vi "PostResults.vi"(0 "reference in":refnum<class "MES_Local.lvclass">, 11 "error in (no error)":errorcluster) -> (4 "reference in":refnum<class "MES_Local.lvclass">, 6 "Status":T1, 15 "error out":errorcluster)   [LabVIEW 2022 SP3, in "MES_Local.lvlib" / "MES_Local.lvclass"]
uses:
  MES_Local.lvclass
  Components/MES_Base.lvlibp/Controls/Status.ctl
  Components/MES_Base.lvlibp/MES_Base.lvclass
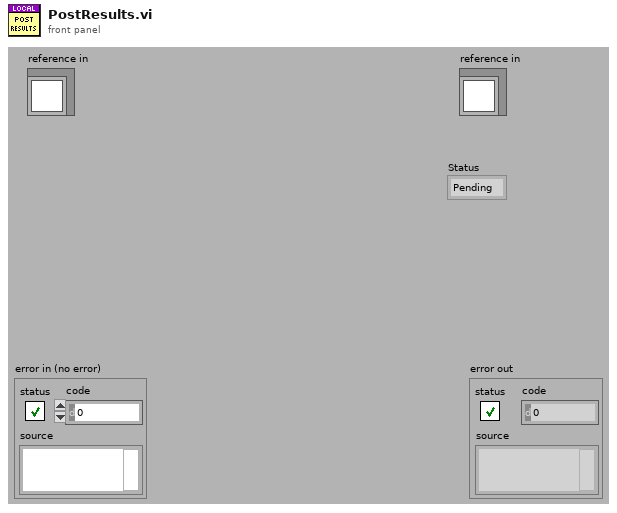
[diagram p1: front panel]
types:
  T1 = typedef "MES_Base.lvlibp/MES_Base.lvclass/Status.ctl" = enum16{"Pending", "Pass", "Fail"}
  T2 = typedef "MES_Local.lvlib/MES_Local.lvclass/ObjectAttributes.ctl" = cluster{"Config":T3, "Logged_In?":bool, "AttributeNames":string[], "AttributeWritten":bool[], "ComponentNames":string[], "TestIndex":i32, "TestTag":string[], "Time Stamp":timestamp, "Employee":string, "Resource_Key":string, "Local Spec":path, "Login":refnum<class "Login_Base.lvclass">, "ReportPath":path, "Spec":T4, "StartTime":timestamp, "Role":string}
  T3 = typedef "MES_Local.lvlib/MES_Local.lvclass/Config.ctl" = cluster{"Results_Path":path}
  T4 = typedef "MES_Base.lvlibp/MES_Base.lvclass/Spec.ctl" = cluster{"Header":cluster{"Doctype":string, "Checksum":string, "DriverKey":string, "SpecId":string, "TransactionId":string, "AccountId":string, "SpecName":string, "WorkflowStep":string, "SerialNumber":string, "BatchNumber":string, "Status":enum16{"Pending", "Pass", "Fail"}, "Comment":string, "FirstFail":string, "Employee":string, "LocalMachine":string, "ResourceKey":string, "Date":string, "Time":string, "Duration":string, "DUT Position":i32}, "Components":cluster{"SerialNumber":string, "PartNumber":string, "Revision":string, "BatchNumber":string, "Name":string, "Description":string, "Attached":bool}[], "Attributes":cluster{"Name":string, "Description":string, "DataType":enum16{"NA", "String", "Boolean", "Int", "Dbl"}, "Value":variant, "DisplayFormat":string, "ReadOnly":bool, "Required":bool}[], "Tests":cluster{"Code":string, "Name":string, "Description":string, "Group":string, "IsGroup":bool, "Tag":string, "Method":string, "Parrameter":string, "DataType":enum16{"NA", "String", "Boolean", "Int", "Dbl"}, "Value":variant, "Status":enum16{"Pending", "Pass", "Fail"}, "LimitLo":variant, "LimitHi":variant, "StringMatch":string, "BooleanMatch":bool, "DisplayFormat":string, "Units":string, "TestTime":dbl}[]}
  T5 = cluster{"Code":string, "Name":string, "Description":string, "Group":string, "IsGroup":bool, "Tag":string, "Method":string, "Parrameter":string, "DataType":enum16{"NA", "String", "Boolean", "Int", "Dbl"}, "Value":variant, "Status":enum16{"Pending", "Pass", "Fail"}, "LimitLo":variant, "LimitHi":variant, "StringMatch":string, "BooleanMatch":bool, "DisplayFormat":string, "Units":string, "TestTime":dbl}[]
  T6 = cluster{"SerialNumber":string, "PartNumber":string, "Revision":string, "BatchNumber":string, "Name":string, "Description":string, "Attached":bool}[]
  T7 = cluster{"Name":string, "Description":string, "DataType":enum16{"NA", "String", "Boolean", "Int", "Dbl"}, "Value":variant, "DisplayFormat":string, "ReadOnly":bool, "Required":bool}[]
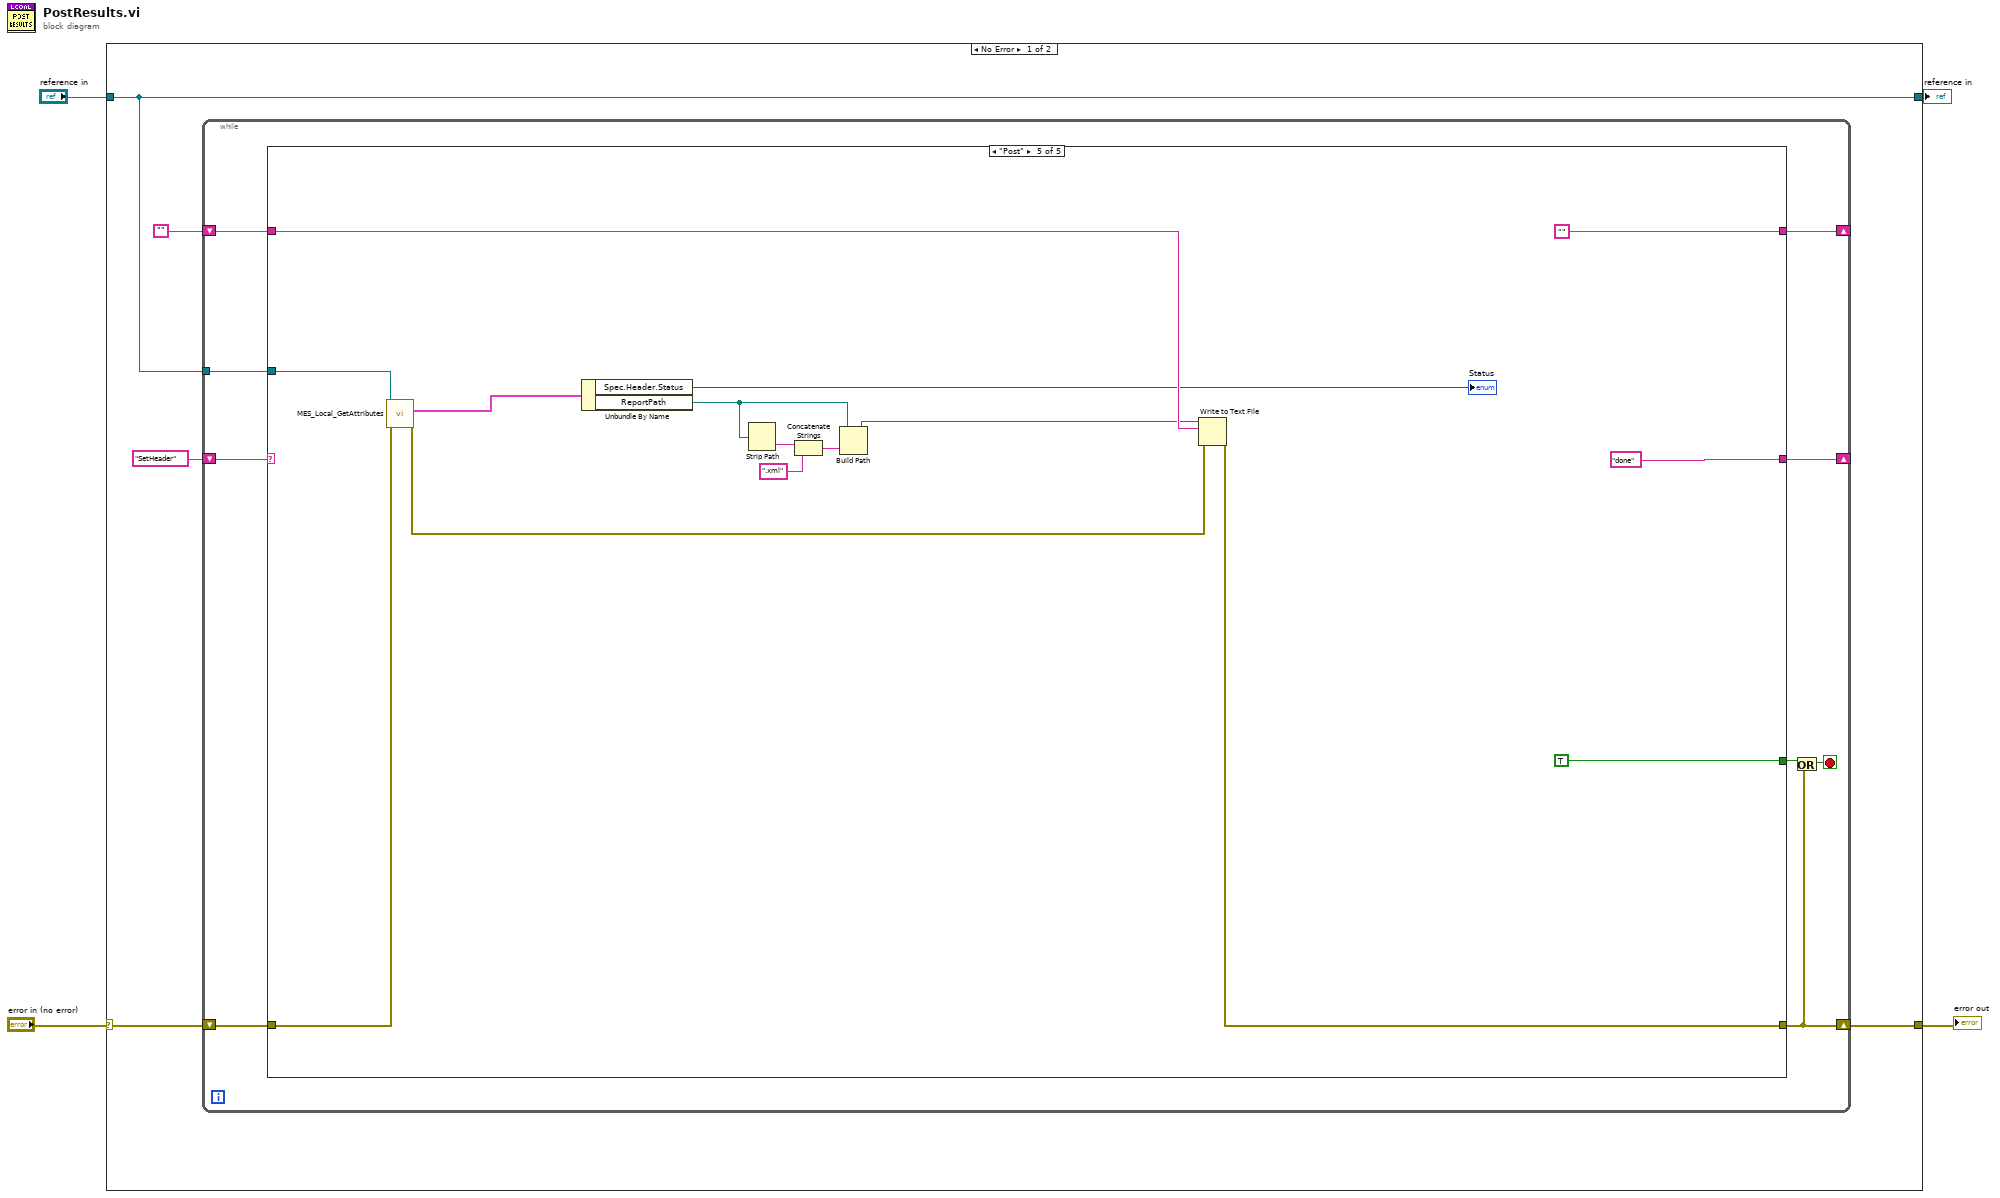
[diagram p0: block diagram]
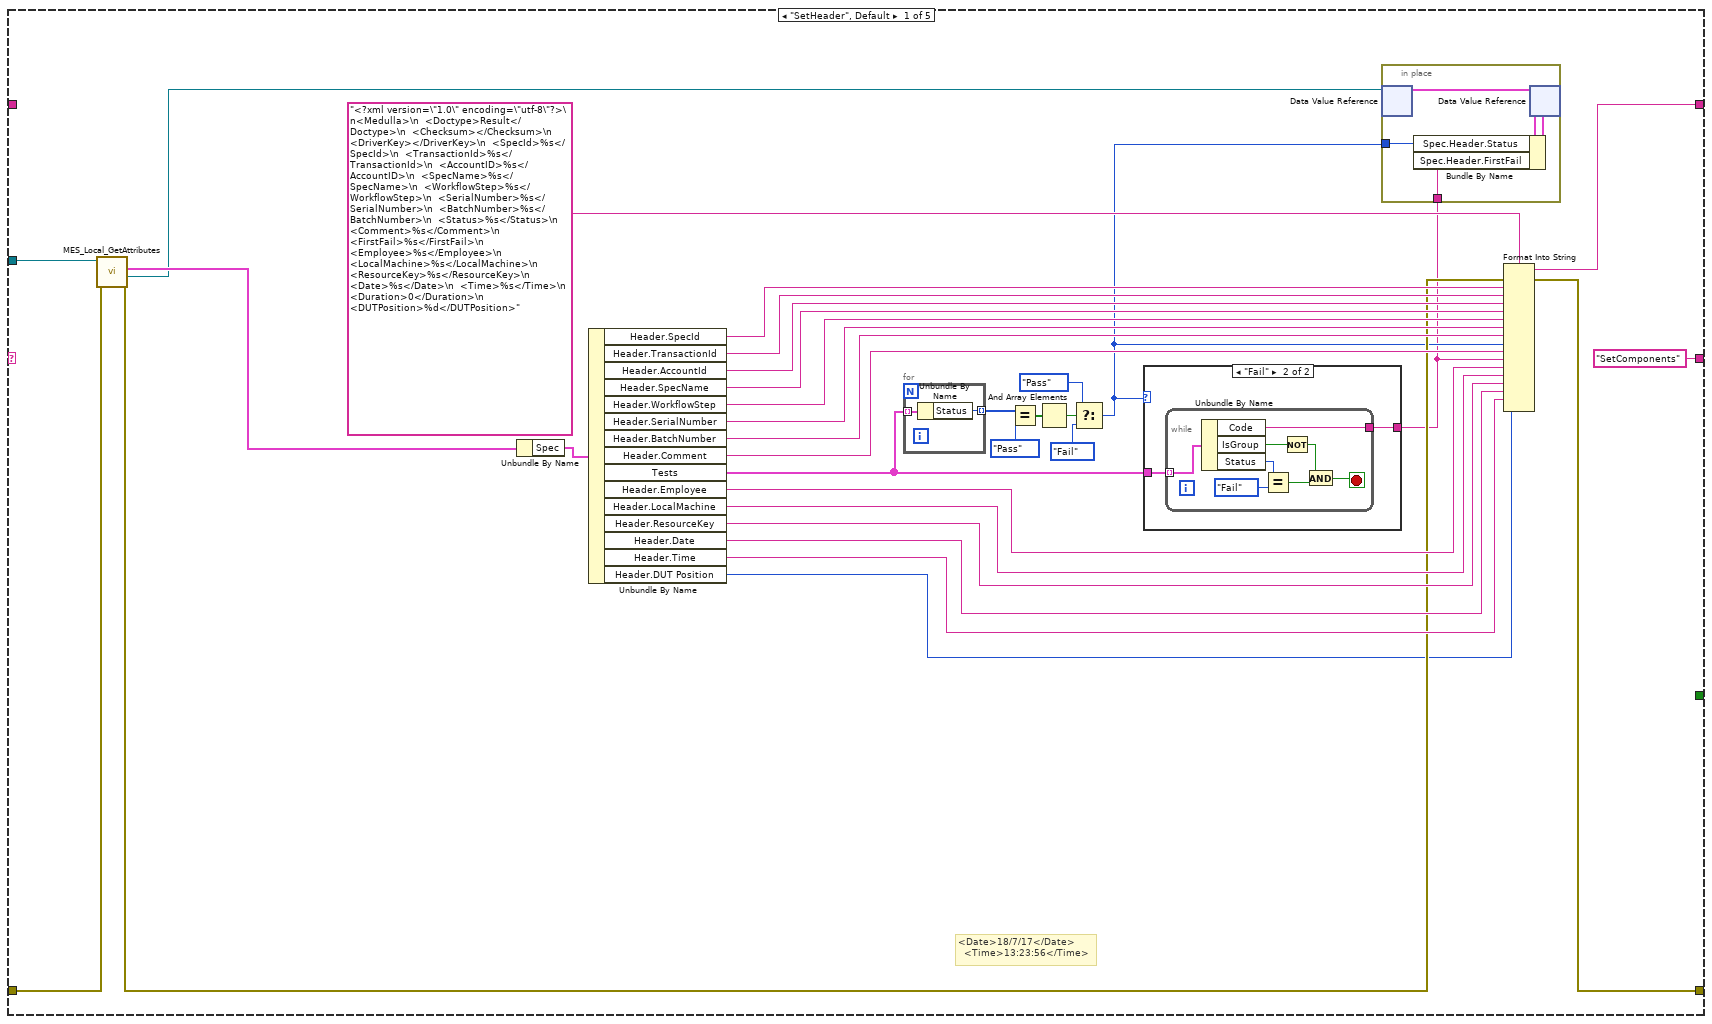
[diagram p2: hidden frame]
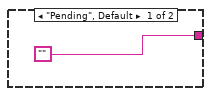
[diagram p3: hidden frame]
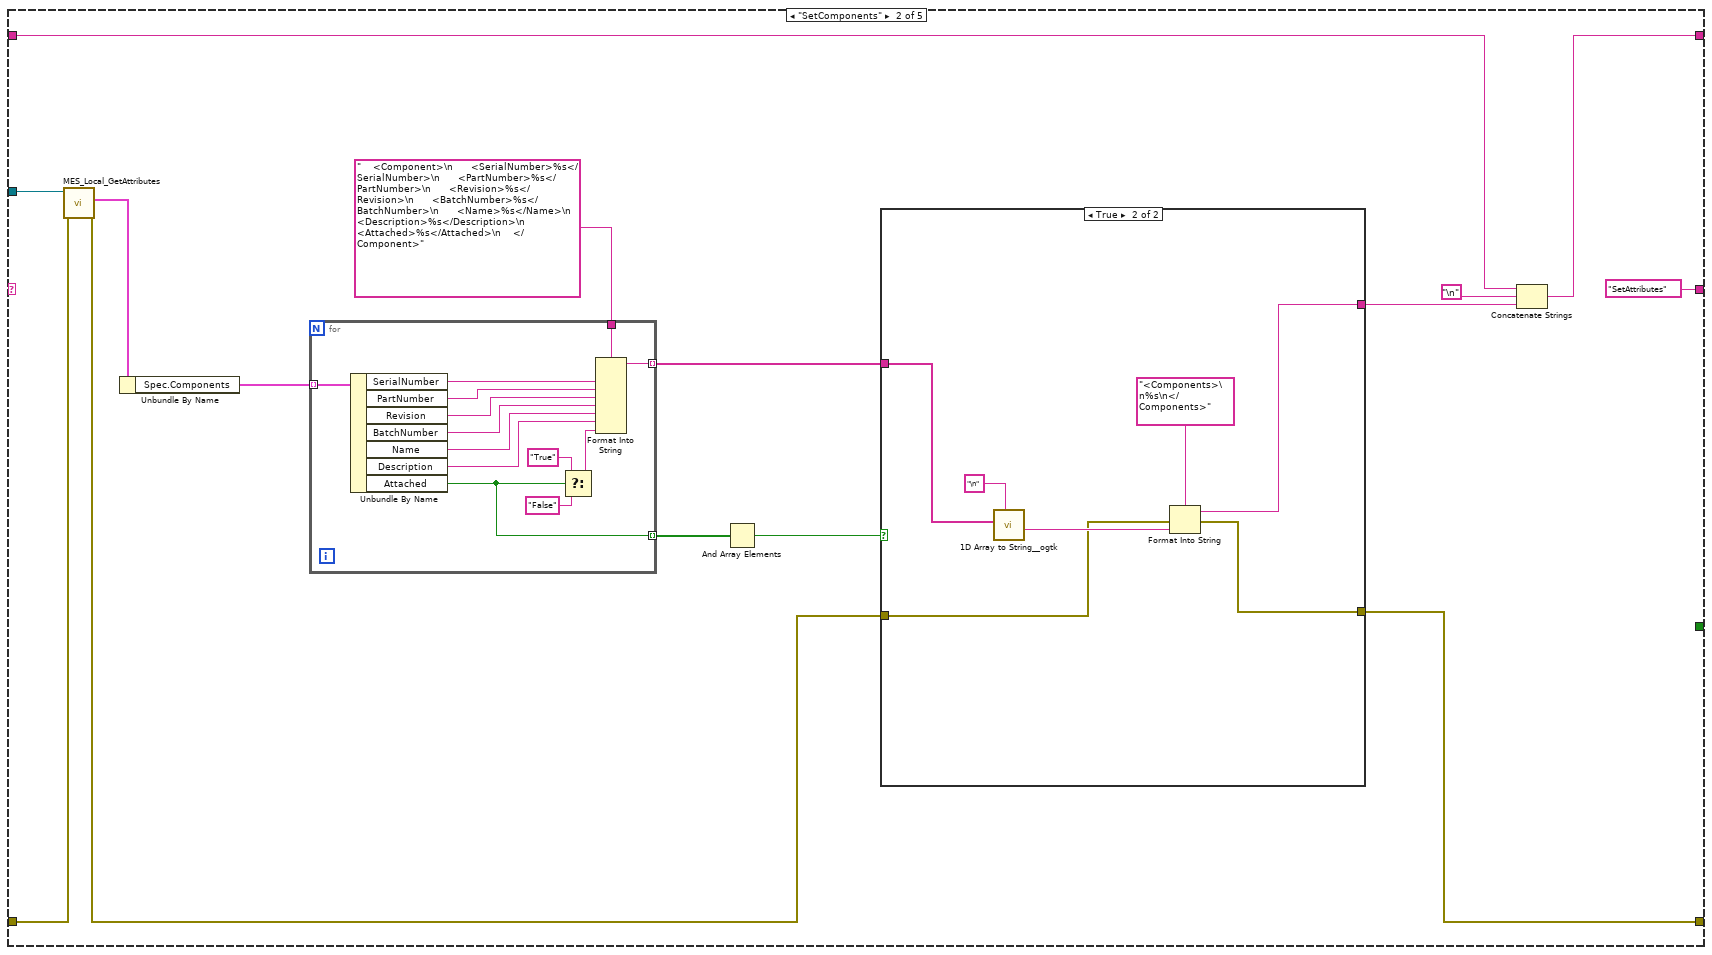
[diagram p4: hidden frame]
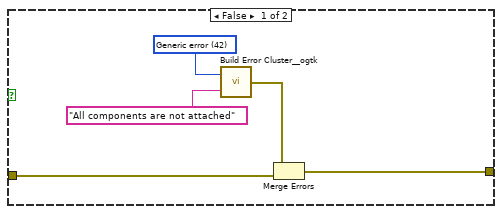
[diagram p5: hidden frame]
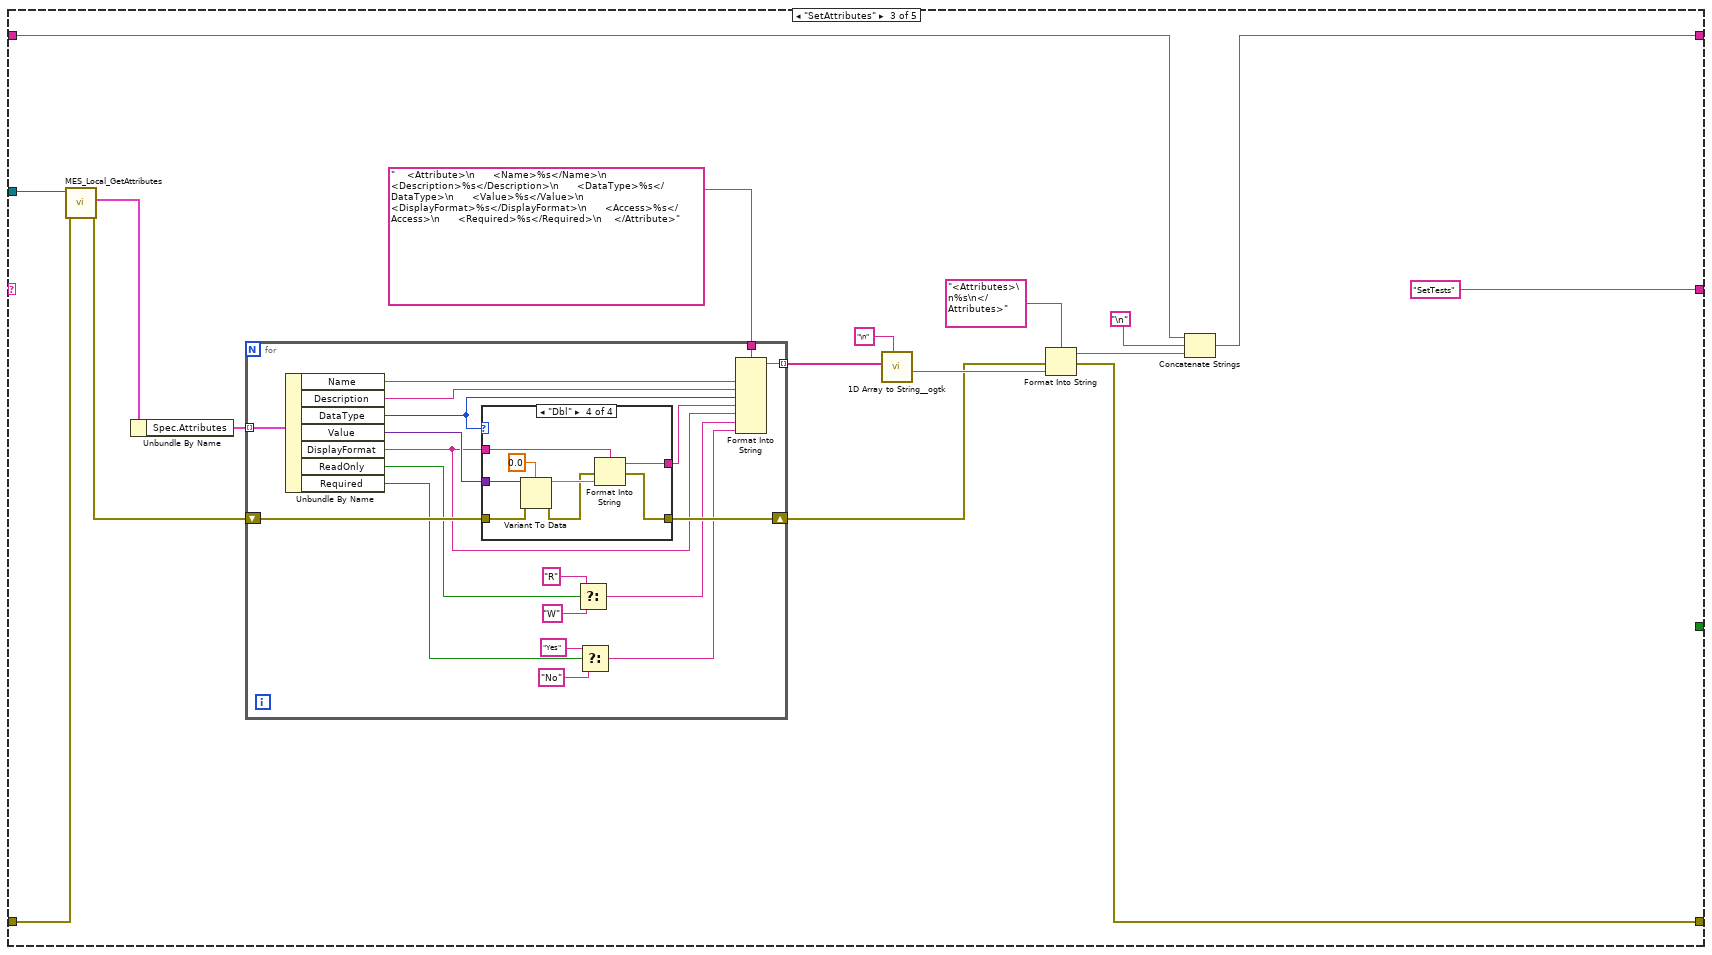
[diagram p6: hidden frame]
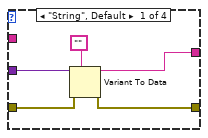
[diagram p7: hidden frame]
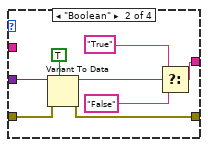
[diagram p8: hidden frame]
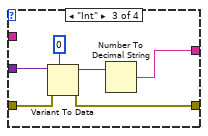
[diagram p9: hidden frame]
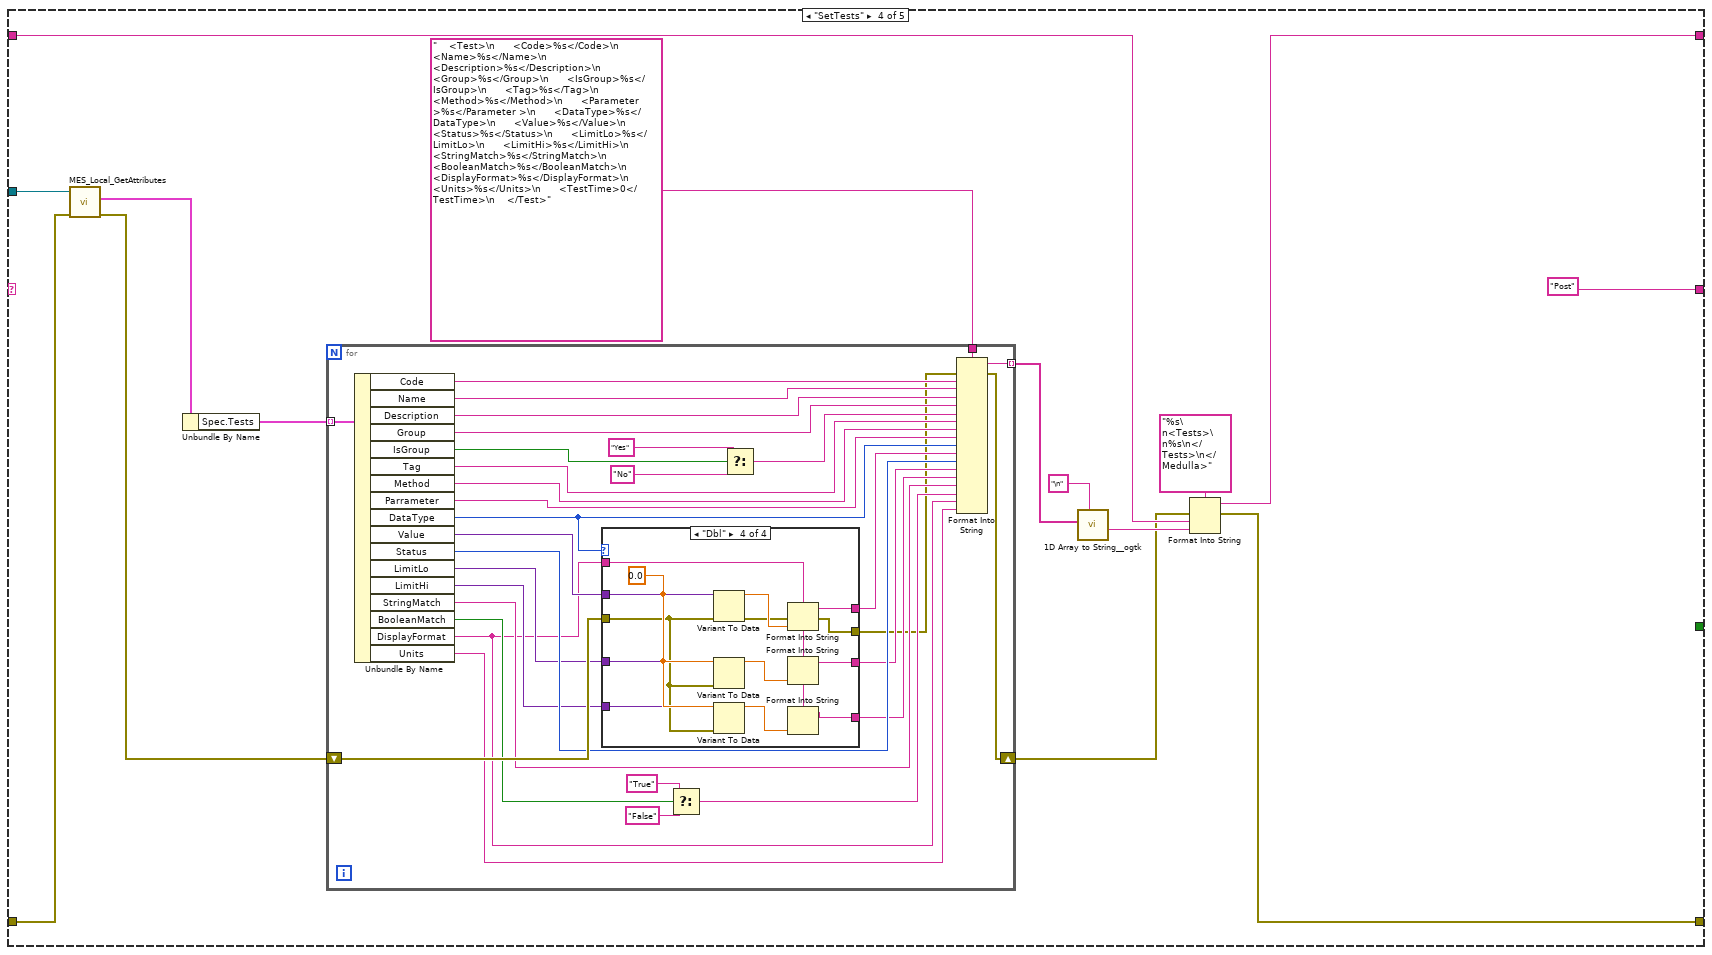
[diagram p10: hidden frame]
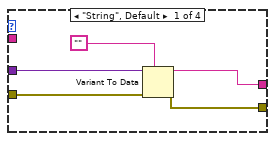
[diagram p11: hidden frame]
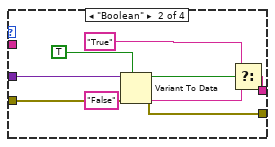
[diagram p12: hidden frame]
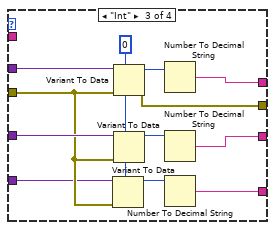
[diagram p13: hidden frame]
diagram:
  n1 = case shown="No Error" "error in (no error)" {
    selector: "error in (no error)" -> [w5 w274]
    tunnel: [w7 w274] -> w3
    tunnel: [w6 w273] -> w1
    tunnel: "reference in" -> [w6 w273]
    frame No Error {
      n2 = while {
        shift-right: [w12] -> _
        shift-left: "SetHeader" -> [w18]
        shift-right: [w16] -> w7
        shift-left: w5 -> [w17]
        shift-right: [w13] -> _
        shift-left: "" -> [w14]
        tunnel: w6 -> [w10]
        stop <- w15 stop-if-true
        n3 = case shown="\"Post\"" w18 {
          tunnel: w17 -> [w28 w71 w111 w173 w267]
          tunnel: [w51 w78 w122 w184 w269] -> w16
          tunnel: w14 -> [_ w76 w117 w183 w268]
          tunnel: [w47 w74 w115 w182 ""] -> w13
          tunnel: ["SetComponents" ("String to Prepend to source (\"\")") "SetAttributes" ("String to Prepend to source (\"\")") "SetTests" ("String to Prepend to source (\"\")") "Post" ("String to Prepend to source (\"\")") "done" ("String to Prepend to source (\"\")")] -> w12
          tunnel: [_ _ _ _ TRUE] -> w11
          tunnel: w10 -> [w29 w72 w112 w175 w266]
          frame "SetHeader", Default {
            # "<Date>18/7/17</Date>\n  <Time>13:23:56</Time>"
            n4 = call "MES_Local_GetAttributes.vi"("error in (no error)"=w28, "reference in"=w29) -> ("error out"=w27:errorcluster, "DataRef"=w25:refnum<data-value>, "Data"=w26:T2)  [unwired: 6 in, 1 out]
            n5 = Unbundle By Name(w26) -> ("Spec"=w48:T4)
            n6 = Unbundle By Name(w48) -> ("Header.SpecId"=w42:string, "Header.TransactionId"=w41:string, "Header.AccountId"=w40:string, "Header.SpecName"=w39:string, "Header.WorkflowStep"=w38:string, "Header.SerialNumber"=w37:string, "Header.BatchNumber"=w36:string, "Header.Comment"=w35:string, "Tests"=w49:T5, "Header.Employee"=w34:string, "Header.LocalMachine"=w33:string, "Header.ResourceKey"=w32:string, "Header.Date"=w31:string, "Header.Time"=w30:string, "Header.DUT Position"=w19:i32)
            n7 = for {
              tunnel: w49 -> [w68] mode=indexing
              tunnel: [w67] -> w50 mode=indexing
              n8 = Unbundle By Name(w68) -> ("Status"=w67:enum16{"Pending", "Pass", "Fail"})
            }
            n9 = Equal?(x=w50, y=Status."Pass" ("Status")) -> (x = y?=w44:bool[])
            n10 = And Array Elements(Boolean array=w44) -> (logical AND=w43:bool)
            n11 = Select(t=Status."Pass" ("Status"), s=w43, f=Status."Fail" ("Status")) -> (s? t:f=w24:T1)
            n12 = case shown="\"Fail\"" w24 {
              tunnel: ["" w57] -> w23
              tunnel: w49 -> [_ w58]
              frame "Pending", Default {
              }
              frame "Fail" {
                n13 = while {
                  tunnel: w58 -> [w66] mode=indexing
                  tunnel: [w60] -> w57
                  stop <- w61 stop-if-true
                  n14 = Unbundle By Name(w66) -> ("Code"=w60:string, "IsGroup"=w65:bool, "Status"=w64:enum16{"Pending", "Pass", "Fail"})
                  n15 = Equal?(x=w64, y=Status."Fail" ("Status")) -> (x = y?=w62:bool)
                  n16 = Not(x=w65) -> (.not. x?=w63:bool)
                  n17 = And(x=w63, y=w62) -> (x .and. y?=w61:bool)
                }
              }
            }
            n18 = in-place {
              in-place-border: w24 -> [w53]
              in-place-border: w23 -> [w52]
              n19 = in-place-dvr #1(w25) -> (w55:T2)  [unwired: 1 out]
              n20 = Bundle By Name(cluster=w55, "Spec.Header.Status"=w53, "Spec.Header.FirstFail"=w52) -> (w54:T2)
              n21 = in-place-dvr #1(w54) -> ()  [unwired: 2 out]
            }
            n22 = Format Into String(format string="<?xml version=\"1.0\" encoding=\"utf-8\"?>\n<Medulla>\n  <Doctype>Result</Doctype>\n  <Checksum></Checksum>\n  <DriverKey></DriverKey>\n  <SpecId>%s</SpecId>\n  <TransactionId>%s</TransactionId>\n  <AccountID>%s</AccountID>\n  <SpecName>%s</SpecName>\n  <WorkflowStep>%s</WorkflowStep>\n  <SerialNumber>%s</SerialNumber>\n  <BatchNumber>%s</BatchNumber>\n  <Status>%s</Status>\n  <Comment>%s</Comment>\n  <FirstFail>%s</FirstFail>\n  <Employee>%s</Employee>\n  <LocalMachine>%s</LocalMachine>\n  <ResourceKey>%s</ResourceKey>\n  <Date>%s</Date>\n  <Time>%s</Time>\n  <Duration>0</Duration>\n <DUTPosition>%d</DUTPosition>", error in=w27, w42, w41, w40, w39, w38, w37, w36, w24, w35, w23, w34, w33, w32, w31, w30, w19) -> (resulting string=w47:string, error out=w51:errorcluster)  [unwired: 1 in]
          }
          frame "SetComponents" {
            n23 = call "MES_Local_GetAttributes.vi"("error in (no error)"=w71, "reference in"=w72) -> ("error out"=w70:errorcluster, "Data"=w69:T2)  [unwired: 6 in, 2 out]
            n24 = Unbundle By Name(w69) -> ("Spec.Components"=w83:T6)
            n25 = for {
              tunnel: w83 -> [w107] mode=indexing
              tunnel: "    <Component>\n      <SerialNumber>%s</SerialNumber>\n      <PartNumber>%s</PartNumber>\n      <Revision>%s</Revision>\n      <BatchNumber>%s</BatchNumber>\n      <Name>%s</Name>\n      <Description>%s</Description>\n      <Attached>%s</Attached>\n    </Component>" -> [w108]
              tunnel: [w97] -> w79 mode=indexing
              tunnel: [w96] -> w81 mode=indexing
              n26 = Unbundle By Name(w107) -> ("SerialNumber"=w106:string, "PartNumber"=w105:string, "Revision"=w104:string, "BatchNumber"=w103:string, "Name"=w102:string, "Description"=w101:string, "Attached"=w96:bool)
              n27 = Select(t="True", s=w96, f="False") -> (s? t:f=w98:string)
              n28 = Format Into String(format string=w108, w106, w105, w104, w103, w102, w101, w98) -> (resulting string=w97:string)  [unwired: 2 in, 1 out]
            }
            n29 = And Array Elements(Boolean array=w81) -> (logical AND=w80:bool)
            n30 = case shown="True" w80 {
              tunnel: w79 -> [_ w94]
              tunnel: w70 -> [w86 w91]
              tunnel: [w85 w90] -> w78
              tunnel: [_ w89] -> w73
              frame False {
                w88 = 42 items=["No error", "Argument error", "Memory is full", "Out of zone", "End of file", "File already open", "Generic file I/O error", "File not found", "File permission error", "Disk is full", "Duplicate path", "Too many files open", "System feature not enabled", "Resource file not found", "Cannot add resource", "Resource not found", "Image not found", "Image memory error", "Pen does not exist", "Config type invalid", "Config token not found", "Config parse error", "Config memory error", "Bad external code format", "Bad external code offset", "External code not present", "Null window", "Destroy window error", "Null menu", "Print aborted", "Bad print record", "Print driver error", "Windows error during printing", "Memory error during printing", "Print dialog error", "Generic print error", "Invalid device refnum", "Device not found", "Device parameter error", "Device unit error", "Cannot open device", "Device call aborted", "Generic error", "Cancelled by user", "Object ID too low", "Object ID too high", "Object not in heap", "Unknown heap", "Unknown object (invalid DefProc)", "Unknown object (DefProc not in table)", "Message out of range", "Invalid (null) method", "Unknown message", "Manager call not supported", "Bad address", "Network operation in progress", "Network operation timed out", "Connection is busy", "Network attribute not supported", "Network error", "Address in use", "System out of memory", "Connection aborted", "Connection refused", "Not connected", "Already connected", "Connection closed", "Initialization error (interapplication manager)", "Bad occurrence", "Wait on unbound occurrence handler", "Occurrence queue overflow", "Datalog type conflict", "Unused", "Unrecognized type (interapplication manager)", "Memory corrupt", "Failed to make temporary DLL", "Old CIN version", "Drag socket not found", "Failed to load drop-object", "Failed to register OLE object", "Failed to release OLE object", "Format specifier type mismatch", "Unknown format specifier", "Too few format specifiers", "Too many format specifiers", "Scan failed", "Newer CIN version", "Error converting to variant", "Runtime menu error", "Password tampered", "Variant attribute not found", "Incompatible variant data type", "Event data is not available", "Event Store is not present", "Occurrence is not found", "Event Queue is not created", "Event info is not available", "Refnum passed is NULL", "Error retrieving Class GUID", "Error retrieving CoClass GUID", "Error retrieving TypeLib GUID.", "Bad built application magic bytes.", "Specific driver is different from the specific driver associated with the Logical Name.", "There is no session opened to the class driver.", "Max Error", "MAX - Error with config objects", "MAX - Error loading configuration", "MAX - Group not supported"]
                n31 = call <userlib>:"Build Error Cluster__ogtk.vi"("String to Prepend to source (\"\")"="All components are not attached" ("String to Prepend to source (\"\")"), "code"=w88) -> ("error out"=w87:errorcluster)
                n32 = Merge Errors(w87, w86) -> (w85:errorcluster)
              }
              frame True {
                n33 = call <userlib>:"1D Array to String__ogtk.vi"("delimiter (Tab)"="\n", "Array of Strings"=w94) -> ("delimited string"=w92:string)  [unwired: 9 in]
                n34 = Format Into String(format string="<Components>\n%s\n</Components>" ("delimiter (Tab)"), error in=w91, w92) -> (resulting string=w89:string, error out=w90:errorcluster)  [unwired: 1 in]
              }
            }
            n35 = Concatenate Strings(w76, "\n", w73) -> (w74:string)
          }
          frame "SetAttributes" {
            n36 = call "MES_Local_GetAttributes.vi"("error in (no error)"=w111, "reference in"=w112) -> ("error out"=w110:errorcluster, "Data"=w109:T2)  [unwired: 6 in, 2 out]
            n37 = Unbundle By Name(w109) -> ("Spec.Attributes"=w125:T7)
            n38 = for {
              tunnel: w125 -> [w143] mode=indexing
              tunnel: "    <Attribute>\n      <Name>%s</Name>\n      <Description>%s</Description>\n      <DataType>%s</DataType>\n      <Value>%s</Value>\n      <DisplayFormat>%s</DisplayFormat>\n      <Access>%s</Access>\n      <Required>%s</Required>\n    </Attribute>" -> [w144]
              tunnel: [w140] -> w123 mode=indexing
              shift-right: [w136] -> w113
              shift-left: w110 -> [w137]
              n39 = Unbundle By Name(w143) -> ("Name"=w142:string, "Description"=w141:string, "DataType"=w139:enum16{"NA", "String", "Boolean", "Int", "Dbl"}, "Value"=w138:variant, "DisplayFormat"=w126:string, "ReadOnly"=w134:bool, "Required"=w131:bool)
              n40 = case shown="\"Dbl\"" w139 {
                tunnel: w138 -> [w147 w155 w161 w170]
                tunnel: w137 -> [w149 w157 w163 w171]
                tunnel: [w148 w156 w162 w164] -> w136
                tunnel: [w145 w150 w158 w166] -> w135
                tunnel: w126 -> [_ _ _ w167]
                frame "String", Default {
                  n41 = Variant To Data(error in=w149, type="", Variant=w147) -> (data=w145:string, error out=w148:errorcluster)
                }
                frame "Boolean" {
                  n42 = Variant To Data(error in=w157, type=TRUE, Variant=w155) -> (data=w153:bool, error out=w156:errorcluster)
                  n43 = Select(t="True" ("delimiter (Tab)"), s=w153, f="False" ("delimiter (Tab)")) -> (s? t:f=w150:string)
                }
                frame "Int" {
                  n44 = Variant To Data(error in=w163, type=0, Variant=w161) -> (data=w159:i32, error out=w162:errorcluster)
                  n45 = Number To Decimal String(number=w159) -> (decimal integer string=w158:string)  [unwired: 1 in]
                }
                frame "Dbl" {
                  n46 = Variant To Data(error in=w171, type=0.0, Variant=w170) -> (data=w168:dbl, error out=w165:errorcluster)
                  n47 = Format Into String(format string=w167, error in=w165, w168) -> (resulting string=w166:string, error out=w164:errorcluster)  [unwired: 1 in]
                }
              }
              n48 = Select(t="R", s=w134, f="W") -> (s? t:f=w127:string)
              n49 = Select(t="Yes", s=w131, f="No") -> (s? t:f=w128:string)
              n50 = Format Into String(format string=w144, w142, w141, w139, w135, w126, w127, w128) -> (resulting string=w140:string)  [unwired: 2 in, 1 out]
            }
            n51 = call <userlib>:"1D Array to String__ogtk.vi"("delimiter (Tab)"="\n", "Array of Strings"=w123) -> ("delimited string"=w119:string)  [unwired: 9 in]
            n52 = Format Into String(format string="<Attributes>\n%s\n</Attributes>" ("delimiter (Tab)"), error in=w113, w119) -> (resulting string=w114:string, error out=w122:errorcluster)  [unwired: 1 in]
            n53 = Concatenate Strings(w117, "\n", w114) -> (w115:string)
          }
          frame "SetTests" {
            n54 = call "MES_Local_GetAttributes.vi"("error in (no error)"=w173, "reference in"=w175) -> ("error out"=w172:errorcluster, "Data"=w174:T2)  [unwired: 6 in, 2 out]
            n55 = Unbundle By Name(w174) -> ("Spec.Tests"=w186:T5)
            n56 = for {
              tunnel: w186 -> [w217] mode=indexing
              tunnel: "    <Test>\n      <Code>%s</Code>\n      <Name>%s</Name>\n      <Description>%s</Description>\n      <Group>%s</Group>\n      <IsGroup>%s</IsGroup>\n      <Tag>%s</Tag>\n      <Method>%s</Method>\n      <Parameter >%s</Parameter >\n      <DataType>%s</DataType>\n      <Value>%s</Value>\n      <Status>%s</Status>\n      <LimitLo>%s</LimitLo>\n      <LimitHi>%s</LimitHi>\n      <StringMatch>%s</StringMatch>\n      <BooleanMatch>%s</BooleanMatch>\n      <DisplayFormat>%s</DisplayFormat>\n      <Units>%s</Units>\n      <TestTime>0</TestTime>\n    </Test>" ("delimiter (Tab)") -> [w218]
              tunnel: [w215] -> w185 mode=indexing
              shift-right: [w190] -> w176
              shift-left: w172 -> [w202]
              n57 = Unbundle By Name(w217) -> ("Code"=w216:string, "Name"=w214:string, "Description"=w213:string, "Group"=w212:string, "IsGroup"=w211:bool, "Tag"=w207:string, "Method"=w206:string, "Parrameter"=w205:string, "DataType"=w203:enum16{"NA", "String", "Boolean", "Int", "Dbl"}, "Value"=w204:variant, "Status"=w200:enum16{"Pending", "Pass", "Fail"}, "LimitLo"=w199:variant, "LimitHi"=w198:variant, "StringMatch"=w195:string, "BooleanMatch"=w194:bool, "DisplayFormat"=w188:string, "Units"=w187:string)
              n58 = case shown="\"Dbl\"" w203 {
                tunnel: w204 -> [w221 w229 w242 w257]
                tunnel: w202 -> [w223 w231 w238 w249]
                tunnel: [w222 w230 w243 w253] -> w189
                tunnel: [w219 w224 w240 w255] -> w201
                tunnel: w188 -> [_ _ _ w248]
                tunnel: w199 -> [_ _ w239 w251]
                tunnel: w198 -> [_ _ w237 w250]
                tunnel: [_ _ w233 w245] -> w197
                tunnel: [_ _ w232 w244] -> w196
                frame "String", Default {
                  n59 = Variant To Data(error in=w223, type="", Variant=w221) -> (data=w219:string, error out=w222:errorcluster)
                }
                frame "Boolean" {
                  n60 = Variant To Data(error in=w231, type=TRUE, Variant=w229) -> (data=w227:bool, error out=w230:errorcluster)
                  n61 = Select(t="True" ("delimiter (Tab)"), s=w227, f="False" ("delimiter (Tab)")) -> (s? t:f=w224:string)
                }
                frame "Int" {
                  w236 = 0
                  n62 = Variant To Data(error in=w238, type=w236, Variant=w237) -> (data=w234:i32)  [unwired: 1 out]
                  n63 = Variant To Data(error in=w238, type=w236, Variant=w242) -> (data=w241:i32, error out=w243:errorcluster)
                  n64 = Variant To Data(error in=w238, type=w236, Variant=w239) -> (data=w235:i32)  [unwired: 1 out]
                  n65 = Number To Decimal String(number=w241) -> (decimal integer string=w240:string)  [unwired: 1 in]
                  n66 = Number To Decimal String(number=w235) -> (decimal integer string=w233:string)  [unwired: 1 in]
                  n67 = Number To Decimal String(number=w234) -> (decimal integer string=w232:string)  [unwired: 1 in]
                }
                frame "Dbl" {
                  w252 = 0.0
                  n68 = Variant To Data(error in=w249, type=w252, Variant=w257) -> (data=w256:dbl, error out=w254:errorcluster)
                  n69 = Variant To Data(error in=w249, type=w252, Variant=w251) -> (data=w247:dbl)  [unwired: 1 out]
                  n70 = Variant To Data(error in=w249, type=w252, Variant=w250) -> (data=w246:dbl)  [unwired: 1 out]
                  n71 = Format Into String(format string=w248, error in=w254, w256) -> (resulting string=w255:string, error out=w253:errorcluster)  [unwired: 1 in]
                  n72 = Format Into String(format string=w248, w247) -> (resulting string=w245:string)  [unwired: 2 in, 1 out]
                  n73 = Format Into String(format string=w248, w246) -> (resulting string=w244:string)  [unwired: 2 in, 1 out]
                }
              }
              n74 = Select(t="True", s=w194, f="False") -> (s? t:f=w191:string)
              n75 = Select(t="Yes", s=w211, f="No") -> (s? t:f=w208:string)
              n76 = Format Into String(format string=w218, error in=w189, w216, w214, w213, w212, w208, w207, w206, w205, w203, w201, w200, w197, w196, w195, w191, w188, w187) -> (resulting string=w215:string, error out=w190:errorcluster)  [unwired: 1 in]
            }
            n77 = call <userlib>:"1D Array to String__ogtk.vi"("delimiter (Tab)"="\n", "Array of Strings"=w185) -> ("delimited string"=w178:string)  [unwired: 9 in]
            n78 = Format Into String(format string="%s\n<Tests>\n%s\n</Tests>\n</Medulla>" ("delimiter (Tab)"), error in=w176, w183, w178) -> (resulting string=w182:string, error out=w184:errorcluster)  [unwired: 1 in]
          }
          frame "Post" {
            n79 = call "MES_Local_GetAttributes.vi"("error in (no error)"=w267, "reference in"=w266) -> ("error out"=w264:errorcluster, "Data"=w265:T2)  [unwired: 6 in, 2 out]
            n80 = Unbundle By Name(w265) -> ("Spec.Header.Status"=→"Status":enum16{"Pending", "Pass", "Fail"}, "ReportPath"=w263:path)
            n81 = Strip Path(path=w263) -> (name=w262:string)  [unwired: 1 out]
            n82 = Concatenate Strings(w262, ".xml" ("string")) -> (w260:string)
            n83 = Build Path(base path=w263, name or relative path=w260) -> (appended path=w259:path)
            n84 = Write to Text File(file (use dialog)=w259, text=w268, error in=w264) -> (error out=w269:errorcluster)  [unwired: 1 in, 2 out]
          }
        }
        n85 = Or(x=w11, y=w16) -> (x .or. y?=w15:bool)
      }
    }
    frame Error {
    }
  }
  "error out" <- w3
  "reference in" <- w1
